vi "Ethernet IP Global Strings.vi"() -> ()   [LabVIEW 2011, in "Ethernet IP Custom Device Custom Device.lvlib"]
uses:
  Ethernet IP Custom Device Custom Device.lvlib
panel:
  in  "Path to L5K file":string="Path to L5K file"
  in  "Update Rate":string="Update Rate"
  in  "Tag Name":string="Tag Name"
  in  "Input?":string="Data Type"
  in  "Data Type":string="Data Type"
  in  "Network Path":string="Network Path"
  in  "Timeout":string="Timeout"
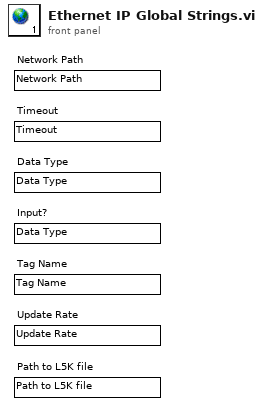
[diagram p1: front panel]
diagram:
